vi "controllerPIP.vi"(8 "error in (no error)":errorcluster) -> (0 "error out":errorcluster)   [LabVIEW 2018]
uses:
  Global_1259.vi
panel:
  out "MTA":bool
  out "RESISTANCE-15":string
  out "INCLINE-14":string
  out "POWER_UP-5, 6":string
  out "FIXTURE_SETUP-1":string
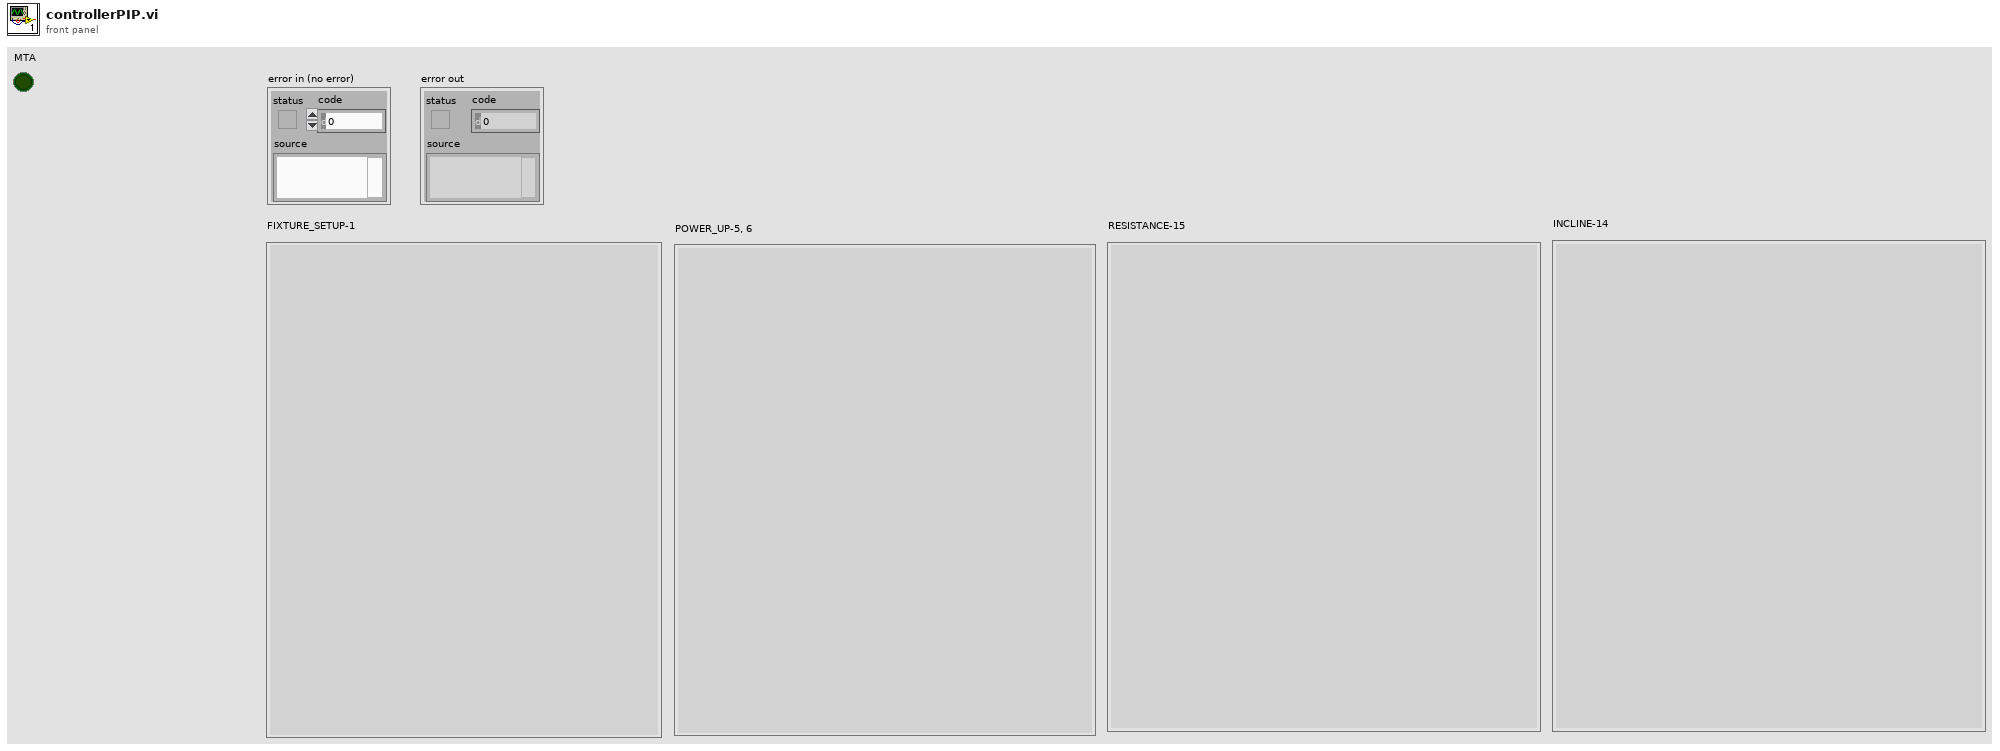
[diagram p1: front panel]
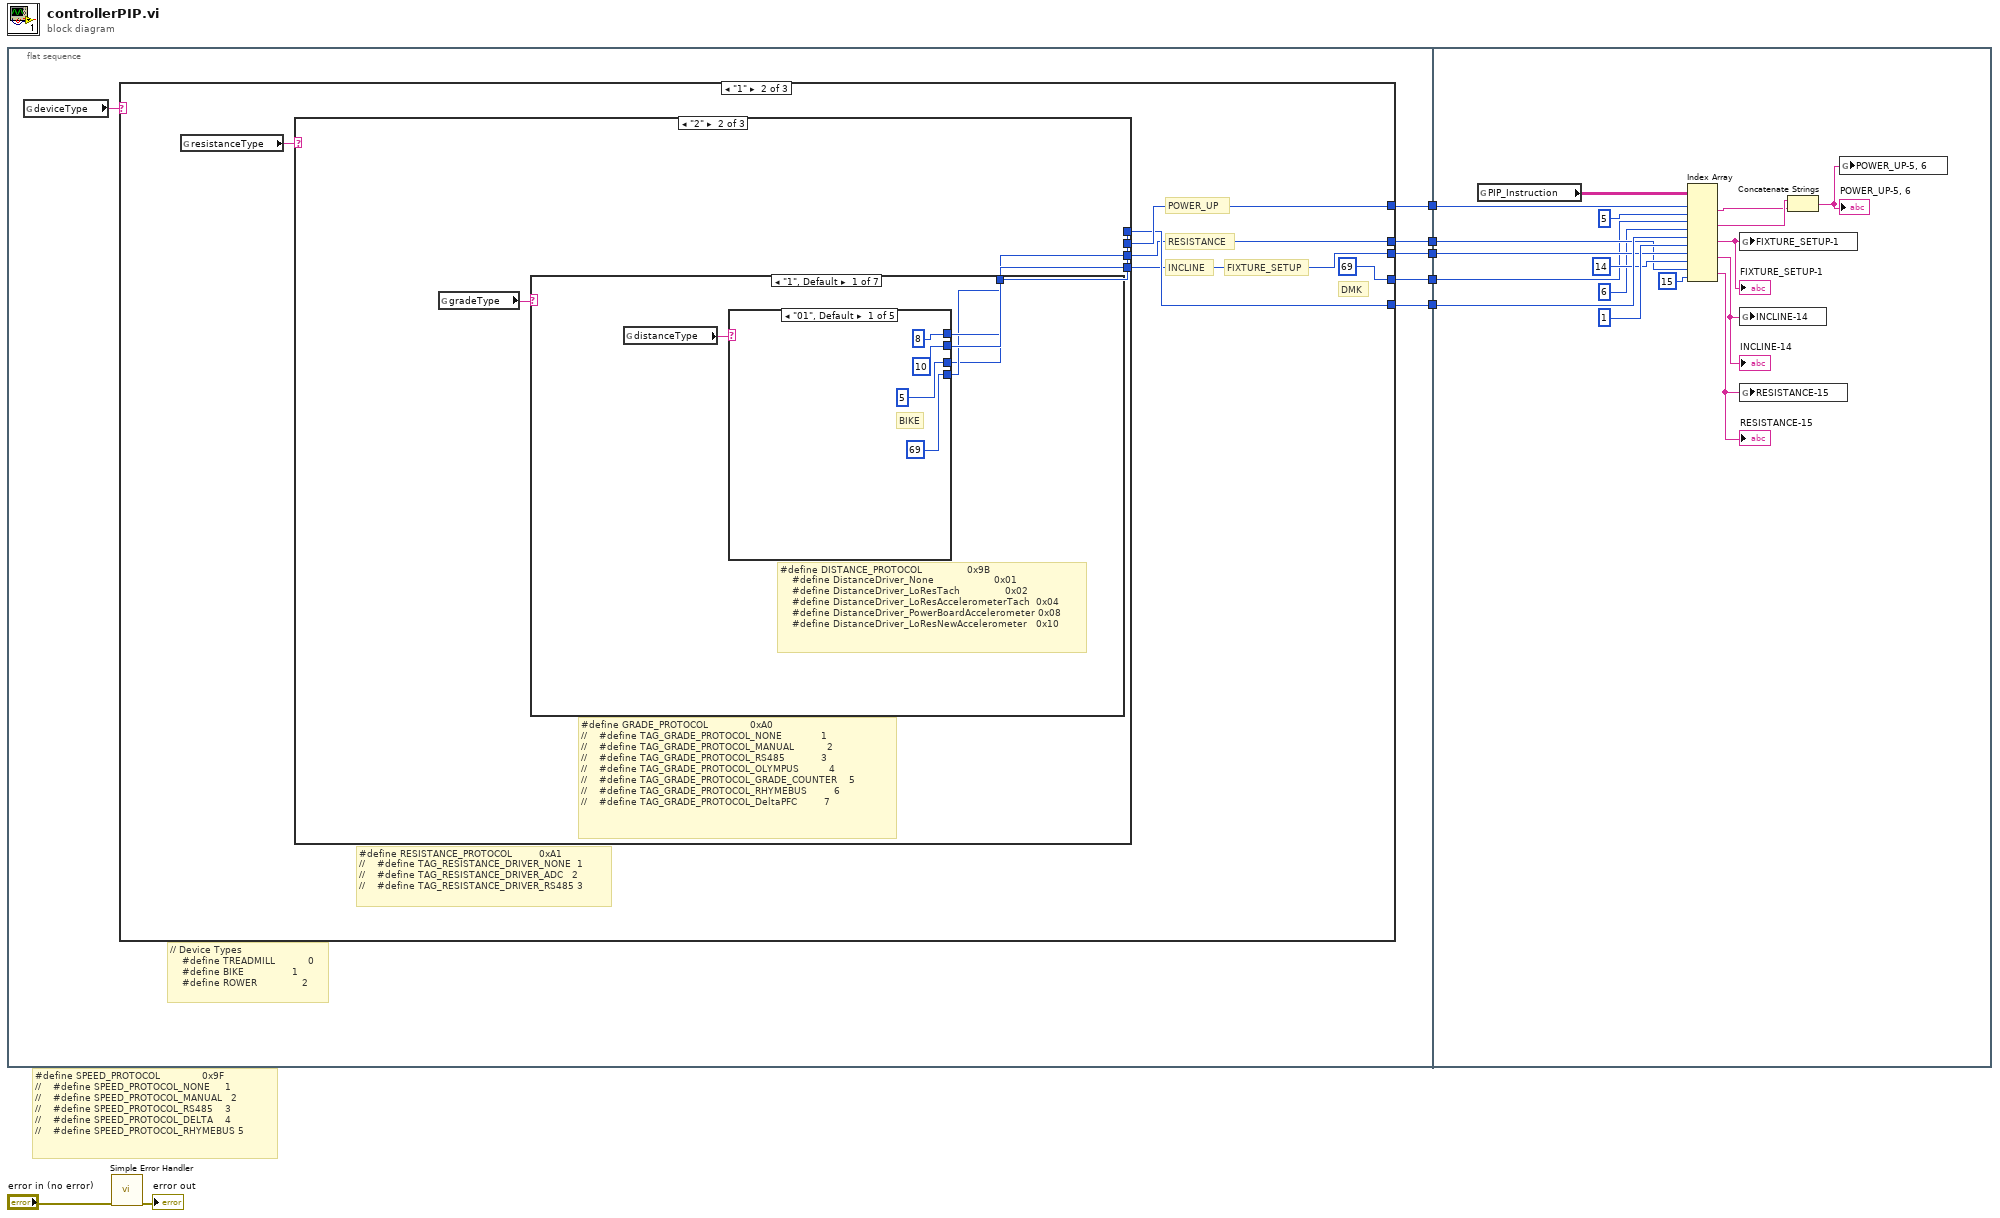
[diagram p0: block diagram]
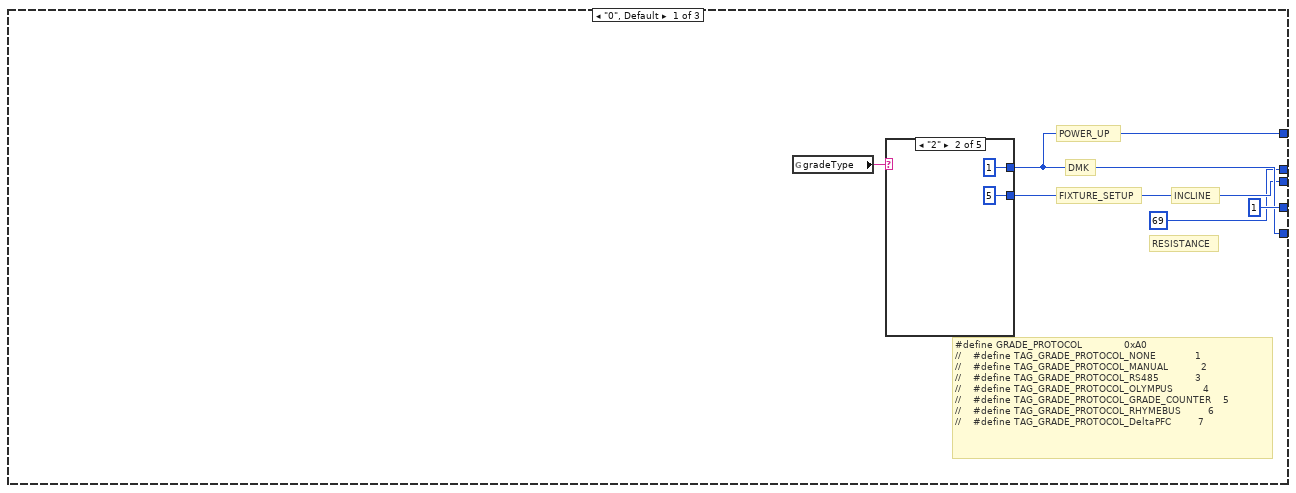
[diagram p2: hidden frame]
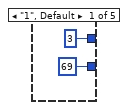
[diagram p3: hidden frame]
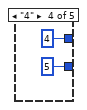
[diagram p5: hidden frame]
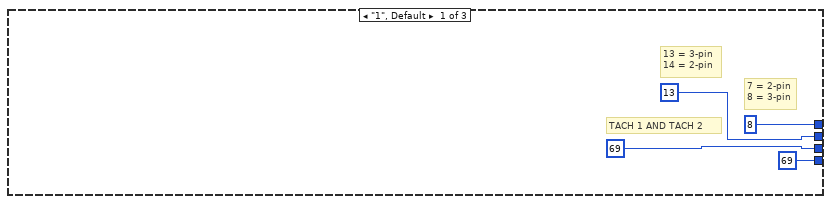
[diagram p7: hidden frame]
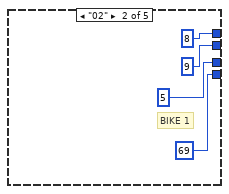
[diagram p8: hidden frame]
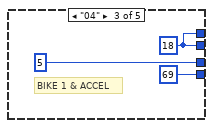
[diagram p9: hidden frame]
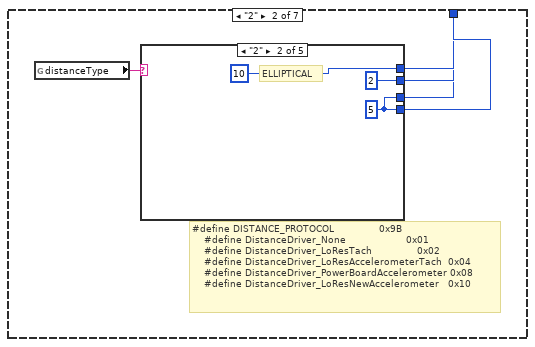
[diagram p12: hidden frame]
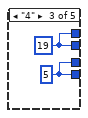
[diagram p14: hidden frame]
diagram:
  # "#define SPEED_PROTOCOL              0x9F\n//    #define SPEED_PROTOCOL_NONE     1\n//    #define SPEED_PROTOCOL_MANUAL   2\n//    #define SPEED_PROTOCOL_RS485    3\n//    #define SPEED_PROTOCOL_DELTA    4\n//    #define SPEED_PROTOCOL_RHYMEBUS 5"
  n1 = flat-sequence {
    tunnel: [w12] -> w7
    tunnel: [w11] -> w6
    tunnel: [w10] -> w5
    tunnel: [w9] -> w2
    tunnel: [w8] -> w1
    tunnel: w7 -> [w147]
    tunnel: w6 -> [w133]
    tunnel: w5 -> [w137]
    tunnel: w2 -> [w144]
    tunnel: w1 -> [w141]
    frame #0 {
      # "// Device Types\n    #define TREADMILL           0\n    #define BIKE                1\n    #define ROWER               2"
      n2 = global read "Global_1259.vi" "deviceType"() -> (w13:string)
      n3 = case shown="\"1\"" w13 {
        tunnel: [w16 w28 w102] -> w12
        tunnel: [1 69 w103] -> w11
        tunnel: [w16 w29 w100] -> w10
        tunnel: [w15 w27 w103] -> w9
        tunnel: [69 w26 w101] -> w8
        frame "0", Default {
          # "RESISTANCE"
          # "#define GRADE_PROTOCOL              0xA0\n//    #define TAG_GRADE_PROTOCOL_NONE             1\n//    #define TAG_GRADE_PROTOCOL_MANUAL           2\n//    #define TAG_GRADE_PROTOCOL_RS485            3\n//    #define TAG_GRADE_PROTOCOL_OLYMPUS          4\n//    #define TAG_GRADE_PROTOCOL_GRADE_COUNTER    5\n//    #define TAG_GRADE_PROTOCOL_RHYMEBUS         6\n//    #define TAG_GRADE_PROTOCOL_DeltaPFC         7"
          # "INCLINE"
          # "FIXTURE_SETUP"
          # "POWER_UP"
          # "DMK"
          n4 = global read "Global_1259.vi" "gradeType"() -> (w18:string)
          n5 = case shown="\"2\"" w18 {
            tunnel: [3 ("t") 1 ("t") _ 4 ("t") _] -> w16
            tunnel: [69 ("t") 5 ("t") _ 5 ("t") _] -> w15
            frame "1", Default {
            }
            frame "2" {
            }
            frame "3" {
            }
            frame "4" {
            }
            frame "5" {
            }
          }
        }
        frame "1" {
          # "#define RESISTANCE_PROTOCOL         0xA1\n//    #define TAG_RESISTANCE_DRIVER_NONE  1\n//    #define TAG_RESISTANCE_DRIVER_ADC   2\n//    #define TAG_RESISTANCE_DRIVER_RS485 3"
          # "POWER_UP"
          # "DMK"
          # "FIXTURE_SETUP"
          # "INCLINE"
          # "RESISTANCE"
          n6 = global read "Global_1259.vi" "resistanceType"() -> (w25:string)
          n7 = case shown="\"2\"" w25 {
            tunnel: [13 w38 w66] -> w29
            tunnel: [8 w37 w67] -> w28
            tunnel: [69 w36 w68] -> w27
            tunnel: [69 w35 w69] -> w26
            frame "1", Default {
              # "TACH 1 AND TACH 2"
              # "7 = 2-pin\n8 = 3-pin"
              # "13 = 3-pin\n14 = 2-pin"
            }
            frame "2" {
              # "#define GRADE_PROTOCOL              0xA0\n//    #define TAG_GRADE_PROTOCOL_NONE             1\n//    #define TAG_GRADE_PROTOCOL_MANUAL           2\n//    #define TAG_GRADE_PROTOCOL_RS485            3\n//    #define TAG_GRADE_PROTOCOL_OLYMPUS          4\n//    #define TAG_GRADE_PROTOCOL_GRADE_COUNTER    5\n//    #define TAG_GRADE_PROTOCOL_RHYMEBUS         6\n//    #define TAG_GRADE_PROTOCOL_DeltaPFC         7"
              n8 = global read "Global_1259.vi" "gradeType"() -> (w39:string)
              n9 = case shown="\"1\", Default" w39 {
                tunnel: [w44 w57 _ _ _ _ _] -> w38
                tunnel: [w43 w58 _ _ _ _ _] -> w37
                tunnel: [w42 w59 _ _ _ _ _] -> w36
                tunnel: [w41 w56 _ _ _ _ _] -> w35
                frame "1", Default {
                  # "#define DISTANCE_PROTOCOL               0x9B\n    #define DistanceDriver_None                    0x01\n    #define DistanceDriver_LoResTach               0x02\n    #define DistanceDriver_LoResAccelerometerTach  0x04\n    #define DistanceDriver_PowerBoardAccelerometer 0x08\n    #define DistanceDriver_LoResNewAccelerometer   0x10"
                  n10 = global read "Global_1259.vi" "distanceType"() -> (w40:string)
                  n11 = case shown="\"01\", Default" w40 {
                    tunnel: [10 9 w55 _ _] -> w44
                    tunnel: [8 8 w55 _ _] -> w43
                    tunnel: [69 69 69 _ _] -> w42
                    tunnel: [5 5 5 _ _] -> w41
                    frame "01", Default {
                      # "BIKE"
                    }
                    frame "02" {
                      # "BIKE 1"
                    }
                    frame "04" {
                      w55 = 18
                      # "BIKE 1 & ACCEL"
                    }
                    frame "08" {
                    }
                    frame "10" {
                    }
                  }
                }
                frame "2" {
                  # "#define DISTANCE_PROTOCOL               0x9B\n    #define DistanceDriver_None                    0x01\n    #define DistanceDriver_LoResTach               0x02\n    #define DistanceDriver_LoResAccelerometerTach  0x04\n    #define DistanceDriver_PowerBoardAccelerometer 0x08\n    #define DistanceDriver_LoResNewAccelerometer   0x10"
                  n12 = global read "Global_1259.vi" "distanceType"() -> (w60:string)
                  n13 = case shown="\"2\"" w60 {
                    tunnel: [_ w61 w64 _ _] -> w59
                    tunnel: [_ 10 w65 _ _] -> w58
                    tunnel: [_ 2 w65 _ _] -> w57
                    tunnel: [_ w61 w64 _ _] -> w56
                    frame "1", Default {
                    }
                    frame "2" {
                      w61 = 5
                      # "ELLIPTICAL"
                    }
                    frame "4" {
                      w64 = 5
                      w65 = 19
                    }
                    frame "8" {
                    }
                    frame "10" {
                    }
                  }
                }
                frame "3" {
                }
                frame "4" {
                }
                frame "5" {
                }
                frame "6" {
                }
                frame "7" {
                }
              }
            }
            frame "3" {
              # "#define GRADE_PROTOCOL              0xA0\n//    #define TAG_GRADE_PROTOCOL_NONE             1\n//    #define TAG_GRADE_PROTOCOL_MANUAL           2\n//    #define TAG_GRADE_PROTOCOL_RS485            3\n//    #define TAG_GRADE_PROTOCOL_OLYMPUS          4\n//    #define TAG_GRADE_PROTOCOL_GRADE_COUNTER    5\n//    #define TAG_GRADE_PROTOCOL_RHYMEBUS         6\n//    #define TAG_GRADE_PROTOCOL_DeltaPFC         7"
              n14 = global read "Global_1259.vi" "gradeType"() -> (w70:string)
              n15 = case shown="\"1\", Default" w70 {
                tunnel: [w75 w88 3 _ _ _ _] -> w66
                tunnel: [w74 w89 11 _ _ _ _] -> w67
                tunnel: [w73 w90 w97 _ _ _ _] -> w68
                tunnel: [w72 w87 w97 _ _ _ _] -> w69
                frame "1", Default {
                  # "#define DISTANCE_PROTOCOL               0x9B\n    #define DistanceDriver_None                    0x01\n    #define DistanceDriver_LoResTach               0x02\n    #define DistanceDriver_LoResAccelerometerTach  0x04\n    #define DistanceDriver_PowerBoardAccelerometer 0x08\n    #define DistanceDriver_LoResNewAccelerometer   0x10"
                  n16 = global read "Global_1259.vi" "distanceType"() -> (w71:string)
                  n17 = case shown="\"01\", Default" w71 {
                    tunnel: [8 9 w86 _ _] -> w75
                    tunnel: [7 8 w86 _ _] -> w74
                    tunnel: [69 69 69 _ _] -> w73
                    tunnel: [5 5 5 _ _] -> w72
                    frame "01", Default {
                      # "BIKE"
                    }
                    frame "02" {
                      # "BIKE 1"
                    }
                    frame "04" {
                      w86 = 18
                      # "BIKE 1 & RS485"
                    }
                    frame "08" {
                    }
                    frame "10" {
                    }
                  }
                }
                frame "2" {
                  # "#define DISTANCE_PROTOCOL               0x9B\n    #define DistanceDriver_None                    0x01\n    #define DistanceDriver_LoResTach               0x02\n    #define DistanceDriver_LoResAccelerometerTach  0x04\n    #define DistanceDriver_PowerBoardAccelerometer 0x08\n    #define DistanceDriver_LoResNewAccelerometer   0x10"
                  n18 = global read "Global_1259.vi" "distanceType"() -> (w91:string)
                  n19 = case shown="\"04\"" w91 {
                    tunnel: [_ w92 w95 _ _] -> w90
                    tunnel: [_ 10 w96 _ _] -> w89
                    tunnel: [_ 2 w96 _ _] -> w88
                    tunnel: [_ w92 w95 _ _] -> w87
                    frame "01", Default {
                    }
                    frame "02" {
                      w92 = 5
                      # "ELLIPTICAL"
                    }
                    frame "04" {
                      w95 = 5
                      w96 = 19
                      # "ELLIPTICAL AND ACCEL"
                    }
                    frame "08" {
                    }
                    frame "10" {
                    }
                  }
                }
                frame "3" {
                  w97 = 5
                  # "RS485"
                }
                frame "4" {
                }
                frame "5" {
                }
                frame "6" {
                }
                frame "7" {
                }
              }
            }
          }
        }
        frame "2" {
          w103 = 69
          # "POWER_UP"
          # "DMK"
          # "FIXTURE_SETUP"
          # "INCLINE"
          # "RESISTANCE"
          n20 = global read "Global_1259.vi" "TABLET"() -> (w104:string)
          n21 = case shown="\"0\", Default" w104 {
            tunnel: [w105 20] -> w102
            tunnel: [w106 5] -> w101
            tunnel: [w107 16] -> w100
            frame "0", Default {
              # "BLE"
              n22 = while {
                tunnel: [w117] -> w108
                stop <- w116 stop-if-true
                n23 = global read "Global_1259.vi" "Part Name"() -> (w115:string)
                n24 = for {
                  tunnel: w115 -> [w129]
                  tunnel: string[] ["59147", "99147", "58118"] -> [w127] mode=indexing
                  tunnel: [w126] -> w118 mode=indexing
                  n25 = Match Pattern(string=w129, regular expression=w127) -> (match substring=w128:string)  [unwired: 1 in, 3 out]
                  n26 = Equal?(x=w127, y=w128) -> (x = y?=w126:bool)
                }
                n27 = while {
                  tunnel: w118 -> [w125]
                  tunnel: [w121] -> w116
                  tunnel: [w120] -> w117
                  i -> [w123]
                  stop <- w121 stop-if-true
                  n28 = Array Size(array=w125) -> (size(s)=w124:i32)
                  n29 = Equal?(x=w123, y=w124) -> (x = y?=w122:bool)
                  n30 = Index Array(array=w125, index=w123) -> (element=w120:bool)
                  n31 = Or(x=w120, y=w122) -> (x .or. y?=w121:bool)
                }
              }
              "MTA" <- w108
              n32 = case shown="True" w108 {
                tunnel: [20 10] -> w107
                tunnel: [1 1] -> w106
                tunnel: [21 8] -> w105
                frame False {
                  # "JST"
                }
                frame True {
                  # "MTA"
                }
              }
            }
            frame "1" {
              # "TABLET"
            }
          }
        }
      }
    }
    frame #1 {
      n33 = global read "Global_1259.vi" "PIP_Instruction"() -> (w136:string[][])
      n34 = Index Array(array=w136, index (row) #1=w137, index (col) #1=5 ("disabled index (col)"), index (row) #2=w133, index (col) #2=6 ("disabled index (col)"), index (row) #3=w147, index (col) #3=1 ("disabled index (col)"), index (row) #4=w144, index (col) #4=14 ("disabled index (col)"), index (row) #5=w141, index (col) #5=15 ("disabled index (col)")) -> (element #1=w134:string, element #2=w135:string, element #3=w146:string, element #4=w143:string, element #5=w140:string)
      "FIXTURE_SETUP-1" <- w146
      "INCLINE-14" <- w143
      "RESISTANCE-15" <- w140
      n35 = global write "Global_1259.vi" "FIXTURE_SETUP-1"(w146) -> ()
      n36 = global write "Global_1259.vi" "INCLINE-14"(w143) -> ()
      n37 = global write "Global_1259.vi" "RESISTANCE-15"(w140) -> ()
      n38 = Concatenate Strings(w135, w134) -> (w149:string)
      "POWER_UP-5, 6" <- w149
      n39 = global write "Global_1259.vi" "POWER_UP-5, 6"(w149) -> ()
    }
  }
  n40 = call <vilib>:"Simple Error Handler.vi"("error in (no error)"="error in (no error)") -> ("error out"=→"error out":errorcluster)  [unwired: 4 in, 4 out]
